vi "ConvertGenericPlotInfo.vi"(11 "GenericPlotOptions in":T1) -> (3 "GenericPlotOptionsOut(NoEnum)":T3)   [LabVIEW 2018, in "LcWebView.lvclass"]
uses:
  LcWebView.lvclass
  plots/ctrls/GenericPlotOption_NoEnumPrivate.ctl
  plots/ctrls/GenericPlotOption.ctl
  plots/ctrls/LegendPosition.ctl
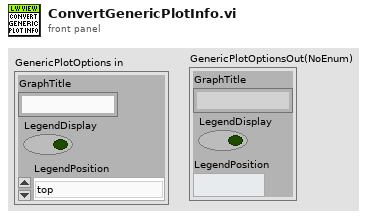
[diagram p1: front panel]
types:
  T1 = typedef "LcWebView.lvclass/GenericPlotOption.ctl" = cluster{"GraphTitle":string, "LegendDisplay":bool, "LegendPosition":T2}
  T2 = typedef "LcWebView.lvclass/LegendPosition.ctl" = enum16{"top", "right", "left", "bottom"}
  T3 = typedef "LcWebView.lvclass/GenericPlotOption_NoEnumPrivate.ctl" = cluster{"GraphTitle":string, "LegendDisplay":bool, "LegendPosition":string}
  T4 = cluster{"GraphTitle":string, "LegendDisplay":bool, "LegendPosition":string}
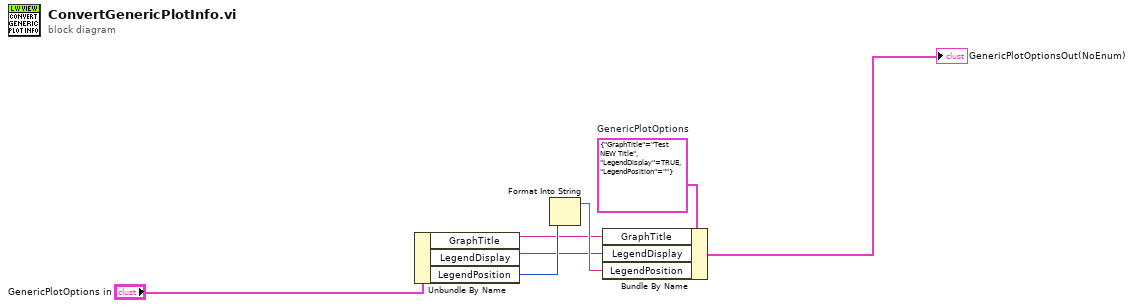
[diagram p0: block diagram]
diagram:
  w2 = T4 {"GraphTitle"="Test NEW Title", "LegendDisplay"=TRUE, "LegendPosition"=""}  # GenericPlotOptions
  n1 = Unbundle By Name("GenericPlotOptions in") -> ("GraphTitle"=w3:string, "LegendDisplay"=w4:bool, "LegendPosition"=w5:T2)
  n2 = Format Into String(w5) -> (resulting string=w6:string)  [unwired: 3 in, 1 out]
  n3 = Bundle By Name(cluster=w2, "GraphTitle"=w3, "LegendDisplay"=w4, "LegendPosition"=w6) -> (→"GenericPlotOptionsOut(NoEnum)":T4)
